vi "testGraph3D.vi"() -> ()   [LabVIEW 2023]
uses:
  <vilib>/Native 3D Graph/xcontrol/3DPC_SurfacePlot.xctl
panel:
  in  "Array 2":dbl[][](array[numeric])
  in  "stop":bool
  in  "Array":dbl[][](array[numeric])
  out "3D Graph":refnum<class "Base Datatype.lvclass">[](xcontrol)
  # "0"
  # "0"
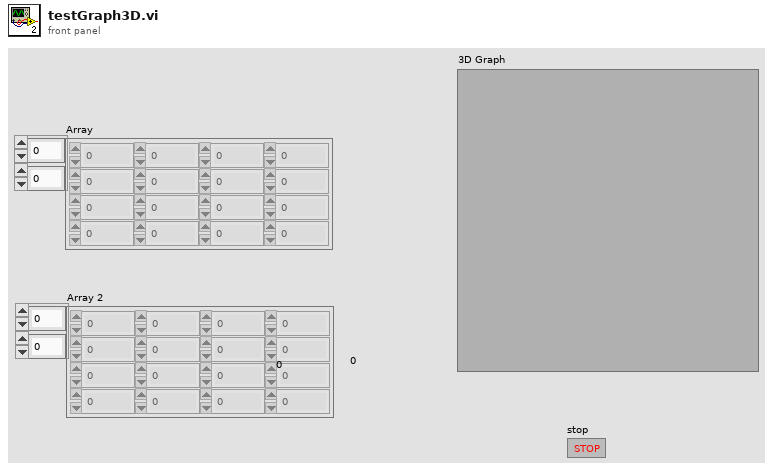
[diagram p1: front panel]
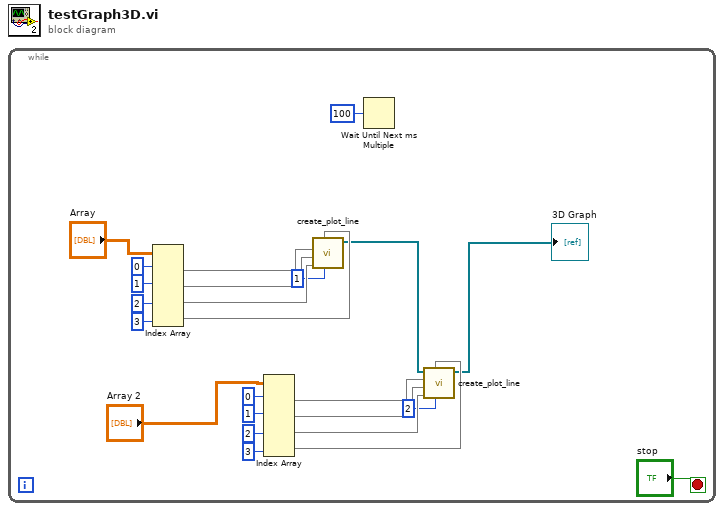
[diagram p0: block diagram]
diagram:
  n1 = while {
    stop <- "stop" stop-if-true
    n2 = Index Array(array="Array", index (row) #1=0 ("index (row)"), index (row) #2=1 ("index (row)"), index (row) #3=2 ("index (row)"), index (row) #4=3 ("index (row)")) -> (element #1=w19:dbl[], element #2=w18:dbl[], element #3=w17:dbl[], element #4=w16:dbl[])  [unwired: 4 in]
    n3 = Index Array(array="Array 2", index (row) #1=0 ("index (row)"), index (row) #2=1 ("index (row)"), index (row) #3=2 ("index (row)"), index (row) #4=3 ("index (row)")) -> (element #1=w10:dbl[], element #2=w11:dbl[], element #3=w12:dbl[], element #4=w13:dbl[])  [unwired: 4 in]
    n4 = call <vilib>:"create_plot_line.vi"("plot ID"=1, "color vector"=w16, "z vector"=w17, "y vector"=w18, "x vector"=w19) -> ("plots out"=w4:refnum<class "Base Datatype.lvclass">[])  [unwired: 1 in, 5 out]
    n5 = Wait Until Next ms Multiple(millisecond multiple=u32 100) -> ()  [unwired: 1 out]
    n6 = call <vilib>:"create_plot_line.vi"("plot ID"=2, "color vector"=w13, "z vector"=w12, "y vector"=w11, "x vector"=w10, "plots in"=w4) -> ("plots out"=→"3D Graph":refnum<class "Base Datatype.lvclass">[])  [unwired: 5 out]
  }
